vi "Draw Depth Frame.vi"(8 "error in (no error)":errorcluster, 10 "U16 Array":u16[](array[numeric]), 11 "Image":T1) -> (0 "error out":errorcluster, 3 "Image Out":T1)   [LabVIEW 2014]
uses:
  <vilib>/vision/Image Controls.llb/IMAQ Image.ctl
  Frame Description FGV [Depth].vi
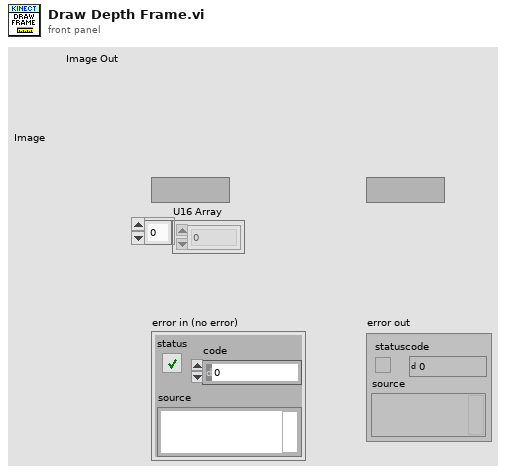
[diagram p1: front panel]
types:
  T1 = typedef "IMAQ Image.ctl" = refnum<image>
  T2 = typedef "FrameDescription.ctl" = cluster{"BytesPerPixel":u32, "DiagonalFieldOfView":sgl, "Height":i32, "HorizontalFieldOfView":sgl, "LengthInPixels":u32, "VerticalFieldOfView":sgl, "Width":i32}
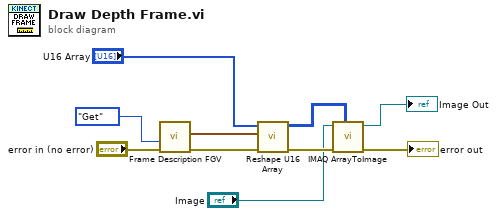
[diagram p0: block diagram]
diagram:
  n1 = call-poly "Frame Description FGV.vi"("error in (no error)"="error in (no error)", "Command"=enum16{"Get", "Set"}."Get") -> ("error out"=w8:errorcluster, "FrameDescription"=w6:T2)  [unwired: 8 in]
  n2 = call "Reshape U16 Array.vi"("error in (no error)"=w8, "FrameDescription"=w6, "U16 Array"="U16 Array") -> ("error out"=w5:errorcluster, "2D Array"=w3:u16[][])  [unwired: 7 in]
  n3 = call "IMAQ ArrayToImage"("Image Pixels (U16)"=w3, "error in (no error)"=w5, "Image"="Image") -> ("error out"=→"error out":errorcluster, "Image Out"=→"Image Out":T1)  [unwired: 7 in]
